vi "CreateCSV.vi"(9 "Data":string, 10 "Append File?":refnum<vi>, 11 "base path":path) -> (3 "path":path)   [LabVIEW 2015]
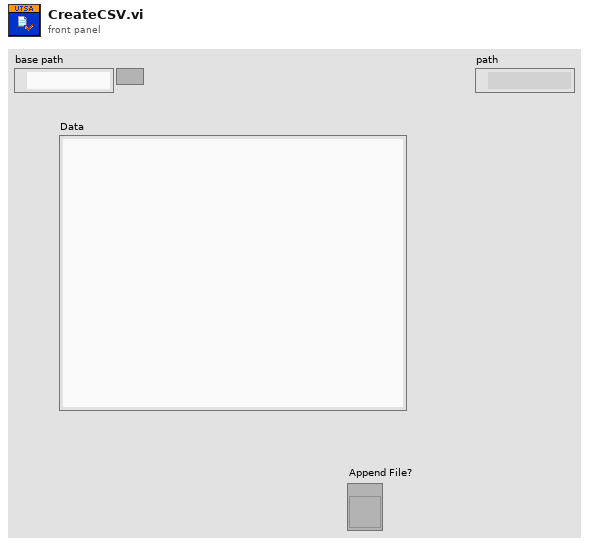
[diagram p1: front panel]
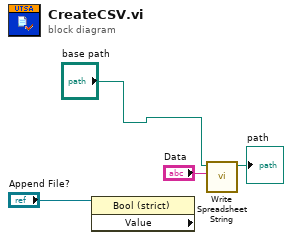
[diagram p0: block diagram]
diagram:
  n1 = property class="Bool (strict)" props=["Value"](reference="Append File?") -> ()  [unwired: 1 in, 3 out]
  n2 = call <vilib>:"Write Spreadsheet String.vi"("spreadsheet string"="Data", "file path (dialog if empty)"="base path") -> ("path"=→"path":path)  [unwired: 8 in, 1 out]
